vi "Unit Test Allow Non-BlueSerializable Objects False.vi"() -> ()   [LabVIEW 2019, in "Sports Unit Tests.lvclass"]
uses:
  Sports Unit Tests.lvclass
  Classes/NonBlueSerializable/NonBlueSerializable.lvclass
  <userlib>/Blue Origin/BlueSerialization/BlueSerializer/SerializeOptions.ctl
  <userlib>/Blue Origin/BlueSerialization/BlueSerializer/DeserializeOptions.ctl
  <userlib>/Blue Origin/BlueSerialization/BlueSerializer/DeserializeSlicingOptions.ctl
  <userlib>/Blue Origin/BlueSerialization/BlueSerializer/DeserializeMutationOptions.ctl
  <userlib>/Blue Origin/BlueSerialization/BlueSerializer/DeserializePreservationOptions.ctl
  <userlib>/Blue Origin/BlueSerialization/BlueSerializer/PreserveNonWiredDataOption.ctl
  Classes/NonBlueSerializable/NonBlueSerializable.lvclass/NonBlueSerializable.ctl
  Classes/NonBlueSerializable/Write Boolean.vi
  Classes/NonBlueSerializable/Write Numeric.vi
  Classes/NonBlueSerializable/Write String.vi
  <vilib>/Utility/error.llb/Clear Errors.vi
  <vilib>/addons/_JKI Toolkits/Caraya/classes/Test/Define Test.vi
  <vilib>/addons/_JKI Toolkits/Caraya/classes/Assert/Assert Equal Value_Variant.vi
  <vilib>/addons/_JKI Toolkits/Caraya/classes/Assert/Assert Error.vi
  <vilib>/addons/_JKI Toolkits/Caraya/classes/Assert/Assert.lvclass
  <userlib>/Blue Origin/BlueSerialization/BlueSerializer/BlueSerializer.lvclass
panel:
  out "Table":string[][](table)
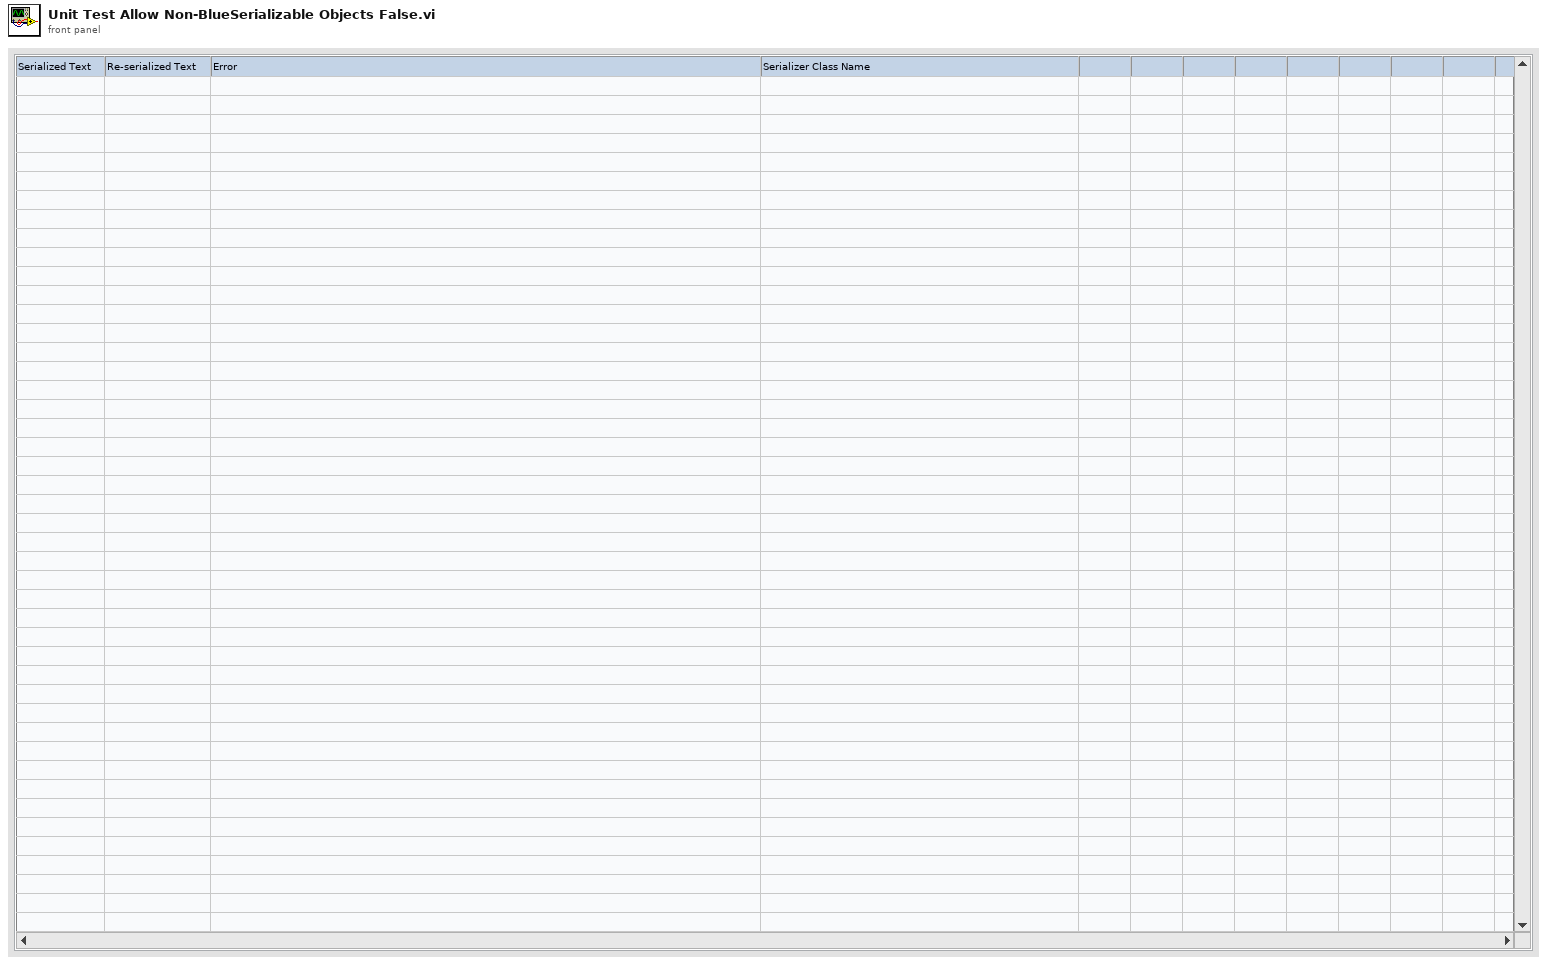
[diagram p1: front panel]
types:
  T1 = typedef "BlueSerialization.lvlib/BlueSerializer.lvclass/DeserializeOptions.ctl" = cluster{"deserialize non-BlueSerializable objects from hex?":bool, "expand objects on type conflict?":bool, "Slicing":T2, "Mutation Options":T3, "Preservation Options":T4}
  T2 = typedef "BlueSerialization.lvlib/BlueSerializer.lvclass/DeserializeSlicingOptions.ctl" = cluster{"slice flattened object data on error?":bool, "sliceable class names":string[]}
  T3 = typedef "BlueSerialization.lvlib/BlueSerializer.lvclass/DeserializeMutationOptions.ctl" = cluster{"error on inserted parent levels?":bool, "\terror on obsolete parent levels?":bool}
  T4 = typedef "BlueSerialization.lvlib/BlueSerializer.lvclass/DeserializePreservationOptions.ctl" = cluster{"Preserve wired serialized data?":bool, "Preserve wired non-serialized data":T5}
  T5 = typedef "BlueSerialization.lvlib/BlueSerializer.lvclass/PreserveNonWiredDataOption.ctl" = enum16{"Don't preserve", "Preserve (error on less-specific wired types)", "Preserve (except on less-specific wired types)"}
  T6 = typedef "BlueSerialization.lvlib/BlueSerializer.lvclass/SerializeOptions.ctl" = cluster{"serialize non-BlueSerializable objects as hex?":bool, "slice objects per SetSerializeSliceClass.vi?":bool}
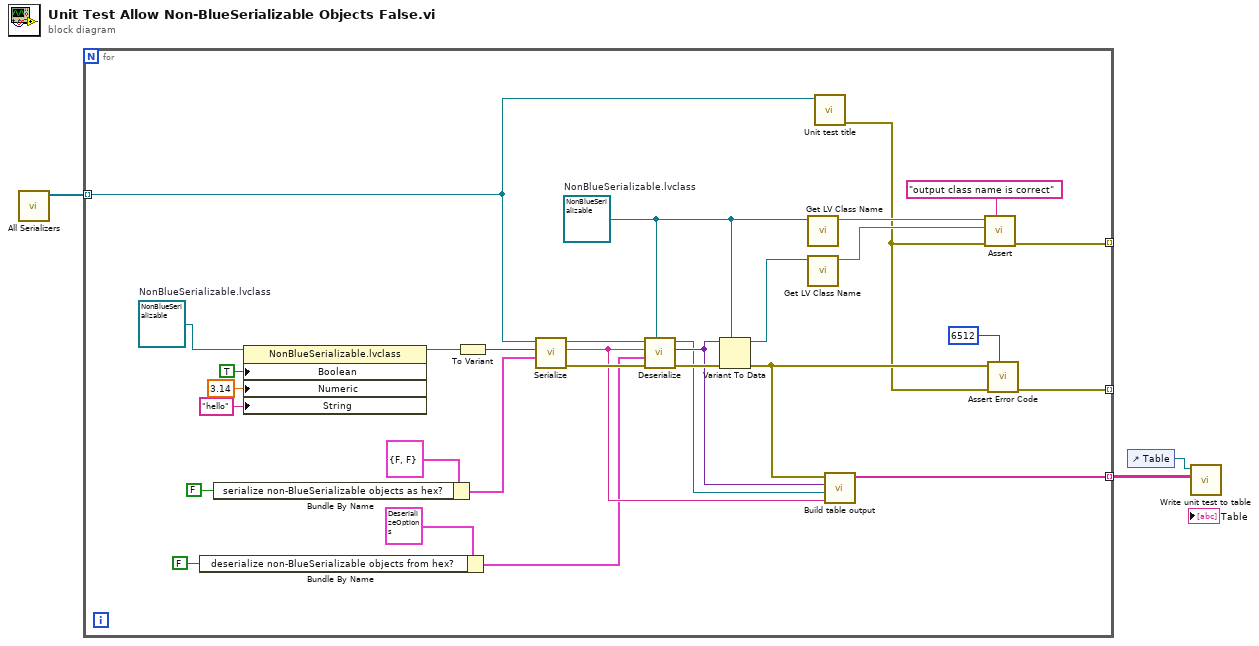
[diagram p0: block diagram]
diagram:
  n1 = call "All Serializers.vi"() -> ("All serializers"=w1:refnum<class "BlueSerializer.lvclass">[])  [unwired: 11 in]
  n2 = for {
    tunnel: w1 -> [w4] mode=indexing
    tunnel: [w18] -> w3 mode=indexing
    tunnel: [w12] -> _ mode=indexing
    tunnel: [w24] -> _ mode=indexing
    w19 = refnum<class "NonBlueSerializable.lvclass"> refnum  # NonBlueSerializable.lvclass
    w23 = refnum<class "NonBlueSerializable.lvclass"> refnum  # NonBlueSerializable.lvclass
    n3 = Bundle By Name(cluster=T1 {"deserialize non-BlueSerializable objects from hex?"=FALSE, "expand objects on type conflict?"=FALSE, "Slicing"={"slice flattened object data on error?"=FALSE, "sliceable class names"=[]}, "Mutation Options"={"error on inserted parent levels?"=FALSE, "\terror on obsolete parent levels?"=FALSE}, "Preservation Options"={"Preserve wired serialized data?"=FALSE, "Preserve wired non-serialized data"=enum."Don't preserve"}} ("Deserialize Options"), "deserialize non-BlueSerializable objects from hex?"=FALSE ("Allow non-BlueSerializable objects?")) -> (w5:T1)
    n4 = Bundle By Name(cluster=T6 {"serialize non-BlueSerializable objects as hex?"=FALSE, "slice objects per SetSerializeSliceClass.vi?"=FALSE} ("Serialize Options"), "serialize non-BlueSerializable objects as hex?"=FALSE ("Allow class slicing?")) -> (w8:T6)
    n5 = property on="Property Node" class="NonBlueSerializable.lvclass"(reference=w23, "Boolean"=TRUE, "Numeric"=3.14, "String"="hello") -> (reference out=w25:refnum<class "NonBlueSerializable.lvclass">)  [unwired: 1 in, 1 out]
    n6 = To Variant(anything=w25) -> (Variant=w31:variant)
    n7 = call <userlib>:"Serialize.vi"("Serialize Options"=w8, "Anything"=w31, "BlueSerializer in"=w4) -> ("error out"=w33:errorcluster, "Serialized Text"=w15:string, "BlueSerializer out"=w32:refnum<class "BlueSerializer.lvclass">)  [unwired: 6 in]
    n8 = call <userlib>:"Deserialize.vi"("Anything"=w19, "error in (no error)"=w33, "Deserialize Options"=w5, "Serialized Text"=w15, "BlueSerializer in"=w32) -> ("error out"=w30:errorcluster, "Variant"=w17:variant, "BlueSerializer out"=w16:refnum<class "BlueSerializer.lvclass">)  [unwired: 4 in]
    n9 = Variant To Data(error in=w30, type=w19, Variant=w17) -> (data=w29:refnum<class "NonBlueSerializable.lvclass">, error out=w14:errorcluster)
    n10 = call <vilib>:"Get LV Class Name.vi"("object"=w19) -> ("class name"=w28:string)  [unwired: 9 in, 1 out]
    n11 = call <vilib>:"Get LV Class Name.vi"("object"=w29) -> ("class name"=w27:string)  [unwired: 9 in, 1 out]
    n12 = call "Unit test title.vi"("serializer"=w4) -> ("error out"=w13:errorcluster)  [unwired: 9 in, 1 out]
    n13 = call "Build table output.vi"("serialized text"=w15, "BlueSerializer in"=w16, "deserialized variant"=w17, "variant to data error"=w14) -> ("table output"=w18:string[])  [unwired: 7 in]
    n14 = call-poly <vilib>:"Assert.vi"("Label"="output class name is correct", "error in (no error)"=w13, "Y"=w27, "X"=w28) -> ("error out"=w24:errorcluster)  [unwired: 7 in]
    n15 = call "Assert Error Code.vi"("Assert specific error code"=6512, "error in (no error)"=w13, "Error?"=w14) -> ("error out"=w12:errorcluster)  [unwired: 8 in]
  }
  n16 = control-ref of="Table"() -> (w2:refnum<vi>)
  n17 = call "Write unit test to table.vi"("Table"=w3, "Table ref in"=w2) -> ()  [unwired: 9 in, 1 out]
